vi "Read TDMS File.vi"(8 "error in (no error)":errorcluster, 11 "Path":path) -> (0 "error out":errorcluster, 3 "Data":dbl[](array[numeric]))   [LabVIEW 2015]
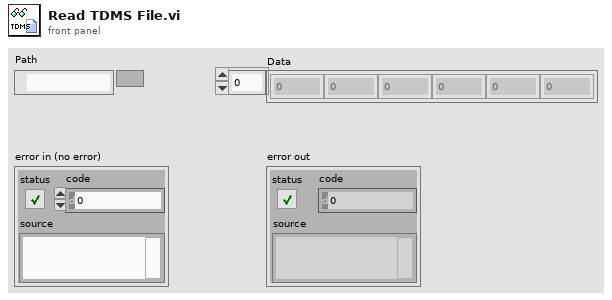
[diagram p1: front panel]
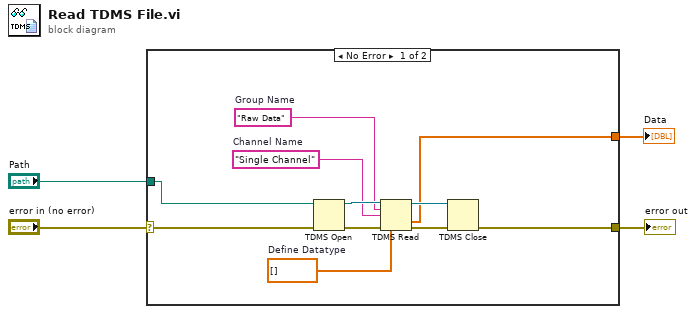
[diagram p0: block diagram]
diagram:
  n1 = case shown="No Error" "error in (no error)" {
    selector: "error in (no error)" -> [w14 w16]
    tunnel: [w13 w16] -> w3
    tunnel: "Path" -> [w15 _]
    tunnel: [w7 _] -> w1
    frame No Error {
      w8 = dbl[] []  # Define Datatype
      w5 = "Single Channel"  # Channel Name
      w6 = "Raw Data"  # Group Name
      n2 = TDMS Open(8:w14, 11:w15) -> (0:w11:errorcluster, 3:w12:refnum<k34>)  [unwired: 5 in]
      n3 = TDMS Read(0:w12, 5:w6, 7:w5, 11:w11, 12:w8) -> (4:w10:refnum<k34>, 10:w7:dbl[], 15:w9:errorcluster)  [unwired: 3 in, 3 out]
      n4 = TDMS Close(8:w9, 11:w10) -> (0:w13:errorcluster)  [unwired: 1 out]
    }
    frame Error {
    }
  }
  "error out" <- w3
  "Data" <- w1
